vi "Get Highest Ver Software By ID.vi"(10 "ID":string, 11 "available software components":T1[](array[typedef]) {"component type" items=["standard", "hidden", "system", "unknown", "startup", "image"]}) -> (2 "found":bool, 3 "Software":T1 {"component type" items=["standard", "hidden", "system", "unknown", "startup", "image"]})   [LabVIEW 2013]
uses:
  <vilib>/nisyscfg/Software 1.2.ctl
  <vilib>/nisyscfg/Component Type.ctl
  <vilib>/nisyscfg/nisyscfg.lvlib
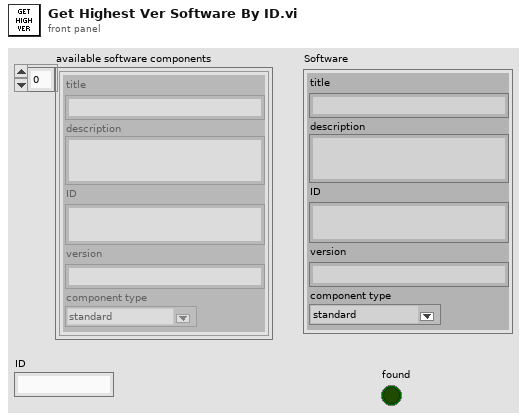
[diagram p1: front panel]
types:
  T1 = typedef "nisyscfg.lvlib/Software 1.2.ctl" = cluster{"title":string, "description":string, "ID":string, "version":string, "component type":T2}
  T2 = typedef "nisyscfg.lvlib/Component Type.ctl" = u32
  T3 = cluster{cluster{i32, i32, i32, i32}, "Software":T1}
  T4 = cluster{cluster{i32, i32, i32, i32}, "Software":T1}[]
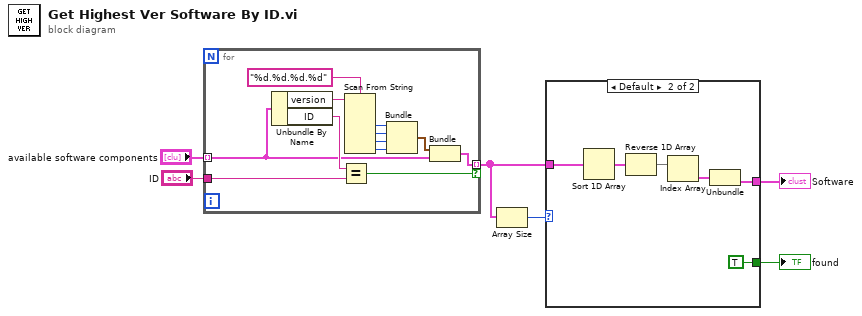
[diagram p0: block diagram]
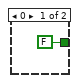
[diagram p2: hidden frame]
diagram:
  n1 = for {
    tunnel: "available software components" -> [w9] mode=indexing
    tunnel: "ID" -> [w17]
    tunnel: [w8] -> w3 mode=indexing if=w7
    n2 = Unbundle By Name(w9) -> ("version"=w11:string, "ID"=w18:string)
    n3 = Equal?(x=w18, y=w17) -> (x = y?=w7:bool)
    n4 = Scan From String(format string="%d.%d.%d.%d", input string=w11) -> (output 1=w13:i32, output 2=w16:i32, output 3=w15:i32, output 4=w14:i32)  [unwired: 6 in, 3 out]
    n5 = Bundle(w13, w16, w15, w14) -> (w10:cluster{i32, i32, i32, i32})  [unwired: 1 in]
    n6 = Bundle(w10, "Software"=w9) -> (w8:T3)  [unwired: 1 in]
  }
  n7 = Array Size(array=w3) -> (size(s)=w2:i32)
  n8 = case shown="Default" w2 {
    tunnel: [_ w25] -> w6
    tunnel: w3 -> [_ w24]
    tunnel: [FALSE TRUE] -> w1
    frame 0 {
    }
    frame Default {
      n9 = Sort 1D Array(array=w24) -> (sorted array=w21:T4)
      n10 = Reverse 1D Array(array=w21) -> (reversed array=w22:T4)
      n11 = Index Array(array=w22) -> (element=w23:T3)  [unwired: 1 in]
      n12 = Unbundle(w23) -> ("Software"=w25:T1)  [unwired: 1 out]
    }
  }
  "Software" <- w6
  "found" <- w1
